vi "Read Controls.vi"(8 "error in (no error)":errorcluster, 11 "Engine in":refnum<class "Engine.lvclass">) -> (0 "error out":errorcluster, 2 "Controls":T1, 3 "Engine out":refnum<class "Engine.lvclass">)   [LabVIEW 2019, in "RT_Game.lvlib" / "Engine.lvclass"]
uses:
  Engine.lvclass
  Game/Controls.ctl
  Game/ControlPlayer.ctl
  Engine.lvclass/Engine.ctl
  Game/Game.lvclass
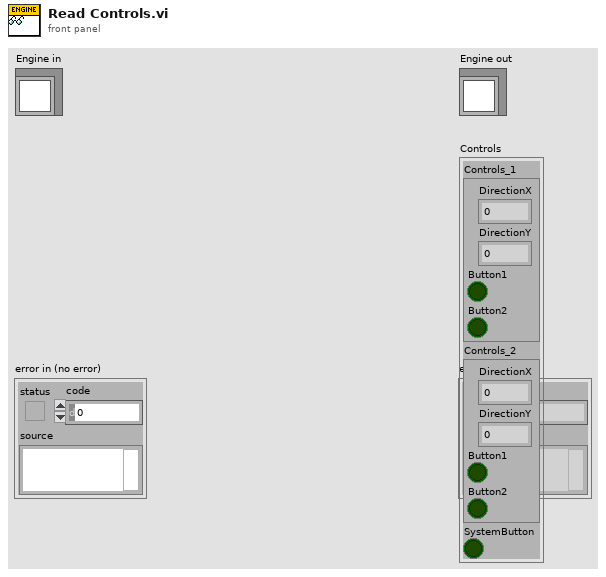
[diagram p1: front panel]
types:
  T1 = typedef "RT_Game.lvlib/Game.lvclass/Controls.ctl" = cluster{"Controls_1":T2, "Controls_2":cluster{"DirectionX":i8, "DirectionY":i8, "Button1":bool, "Button2":bool}, "SystemButton":bool}
  T2 = typedef "RT_Game.lvlib/Game.lvclass/ControlPlayer.ctl" = cluster{"DirectionX":i8, "DirectionY":i8, "Button1":bool, "Button2":bool}
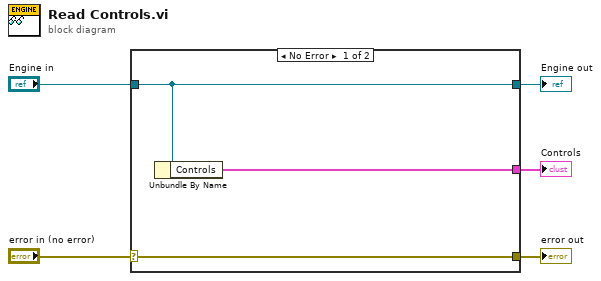
[diagram p0: block diagram]
diagram:
  n1 = case shown="No Error" "error in (no error)" {
    selector: "error in (no error)" -> [w8 w9]
    tunnel: [w8 w9] -> w4
    tunnel: [w7 w10] -> w2
    tunnel: "Engine in" -> [w7 w10]
    tunnel: [w6 _] -> w1
    frame No Error {
      n2 = Unbundle By Name(w7) -> ("Controls"=w6:T1)
    }
    frame Error {
    }
  }
  "error out" <- w4
  "Engine out" <- w2
  "Controls" <- w1
